vi "Insert Important Module VIs.vi"(7 "Application in":refnum<vi>, 8 "Tree Map in":T1, 9 "Root path":string, 10 "DQMH Lib In":refnum<vi>) -> (0 "Tree Map Out":T1)   [LabVIEW 2019, in "Panther Dashboard.lvlib"]
uses:
  Panther Dashboard.lvlib
  <vilib>/National Instruments/Tree Map/Tree Map Data.ctl
  Map Attribute--enum.ctl
  <vilib>/National Instruments/Tree Map/Tree Map.lvlib
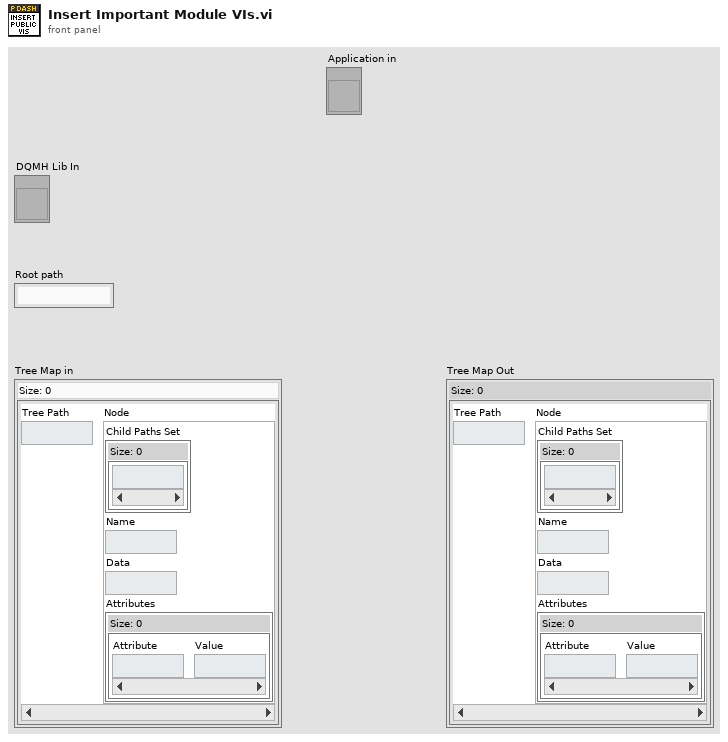
[diagram p1: front panel]
types:
  T1 = typedef "Tree Map.lvlib/Tree Map Data.ctl" = map{string, cluster{"Child Paths Set":set{string}, "Name":string, "Data":string, "Attributes":map{string, string}}}
  T2 = typedef "Panther Dashboard.lvlib/Map Attribute--enum.ctl" = enum16{"Path", "ModuleType", "Module Description", "Dependency?", "Target"}
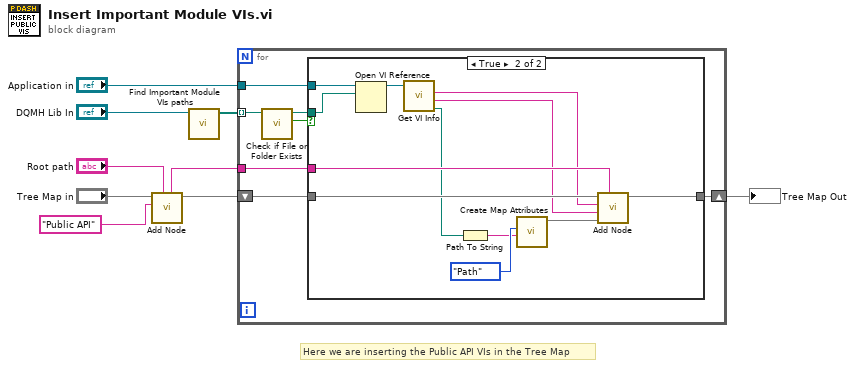
[diagram p0: block diagram]
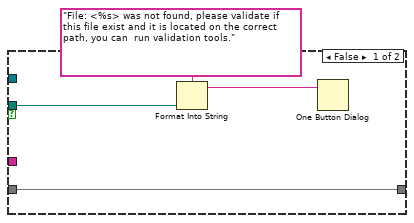
[diagram p2: hidden frame]
diagram:
  # "Here we are inserting the Public API VIs in the Tree Map"
  n1 = call <vilib>:"Add Node.vi"("Parent Path"="Root path", "New Node Name"="Public API", "Tree Map In"="Tree Map in") -> ("Tree Map Out"=w3:T1, "New Node Path"=w1:string)  [unwired: 6 in, 1 out]
  n2 = call "Find Important Module VIs paths.vi"("Library in"="DQMH Lib In") -> ("Public API VIs Paths"=w8:path[])  [unwired: 10 in]
  n3 = for {
    tunnel: "Application in" -> [w16]
    tunnel: w8 -> [w12] mode=indexing
    shift-right: [w15] -> w7
    shift-left: w3 -> [w14]
    tunnel: w1 -> [w13]
    n4 = call <vilib>:"Check if File or Folder Exists.vi"("path"=w12) -> ("file or folder exists?"=w11:bool, "dup path"=w10:path)  [unwired: 8 in, 1 out]
    n5 = case shown="True" w11 {
      tunnel: w16 -> [_ w32]
      tunnel: [w20 w31] -> w15
      tunnel: w14 -> [w20 w30]
      tunnel: w13 -> [_ w29]
      tunnel: w10 -> [w19 w25]
      frame False {
        n6 = Format Into String(format string="File: <%s> was not found, please validate if this file exist and it is located on the correct path, you can  run validation tools.", w19) -> (resulting string=w18:string)  [unwired: 2 in, 1 out]
        n7 = One Button Dialog(message=w18) -> ()  [unwired: 1 in, 1 out]
      }
      frame True {
        n8 = Open VI Reference(application reference (local)=w32, vi path=w25) -> (vi reference=w27:refnum<vi>)  [unwired: 4 in, 1 out]
        n9 = call "Get VI Info.vi"("VI in"=w27) -> ("VI Path"=w21:path, "Full Vi Name"=w26:string, "Plain Name"=w28:string)  [unwired: 7 in, 1 out]
        n10 = Path To String(path=w21) -> (string=w23:string)
        n11 = call "Create Map Attributes.vi"("Attribute"=w23, "Map Attribute"=Map_Attribute--enum."Path") -> ("Root Attributes"=w22:map{string, string})  [unwired: 9 in]
        n12 = call <vilib>:"Add Node.vi"("Parent Path"=w29, "Attributes"=w22, "Data"=w26, "New Node Name"=w28, "Tree Map In"=w30) -> ("Tree Map Out"=w31:T1)  [unwired: 4 in, 2 out]
      }
    }
  }
  "Tree Map Out" <- w7
